vi "BLPop.vi"(0 "reference in":refnum<class "Redis.lvclass">, 1 "Key":string, 7 "Count":u32, 11 "Error In":errorcluster, 13 "Timeout(1000ms)":i32=1000) -> (4 "reference out":refnum<class "Redis.lvclass">, 8 "Elements":string[](array[string]), 15 "Error Out":errorcluster)   [LabVIEW 2020, in "Redis.lvclass"]
doc: "<b>BLPOP</b>\n\nBLPOP is a blocking list pop primitive. It is the blocking version of LPOP because it blocks the connection when there are no elements to pop from any of the given lists. An element is popped from the head of the first list that is non-empty, with the given keys being checked in the order that they are given."
uses:
  Redis.lvclass
  Redis.lvclass/Redis.ctl
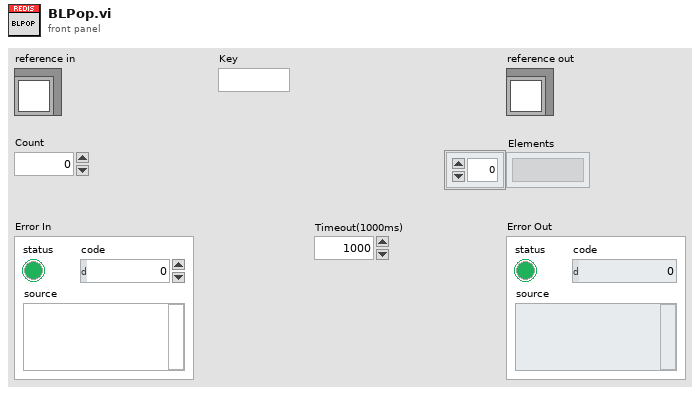
[diagram p1: front panel]
types:
  T1 = typedef "Redis.lvclass/RedisDataType.ctl" = cluster{"Reply Type":T2, "Integer":i64, "String":string, "Multibulk":variant[], "StringData":string[]}
  T2 = typedef "Redis.lvclass/ReplyDataTypeEnum.ctl" = enum16{"None", "Error", "Status", "Nil", "Integer", "String", "Multibulk"}
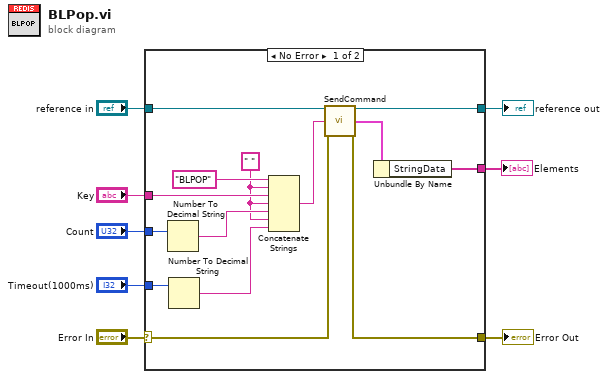
[diagram p0: block diagram]
diagram:
  n1 = case shown="No Error" "Error In" {
    selector: "Error In" -> [w20 w24]
    tunnel: [w19 w24] -> w7
    tunnel: [w22 w23] -> w5
    tunnel: "reference in" -> [w21 w23]
    tunnel: "Key" -> [w17 _]
    tunnel: [w14 _] -> w3
    tunnel: "Count" -> [w13 _]
    tunnel: "Timeout(1000ms)" -> [w9 _]
    frame No Error {
      w11 = " "
      n2 = Number To Decimal String(number=w13) -> (decimal integer string=w12:string)  [unwired: 1 in]
      n3 = Number To Decimal String(number=w9) -> (decimal integer string=w10:string)  [unwired: 1 in]
      n4 = Concatenate Strings("BLPOP", w11, w17, w11, w12, w11, w10) -> (w16:string)
      n5 = call "SendCommand.vi"("reference in"=w21, "Command"=w16, "Error In"=w20) -> ("reference out"=w22:refnum<class "Redis.lvclass">, "Data"=w15:T1, "Error Out"=w19:errorcluster)  [unwired: 10 in]
      n6 = Unbundle By Name(w15) -> ("StringData"=w14:string[])
    }
    frame Error {
    }
  }
  "Error Out" <- w7
  "reference out" <- w5
  "Elements" <- w3
